vi "Requests.vi"(8 "error in (no error)":errorcluster, 9 "write enable":bool=TRUE, 11 "ICPCON ET7028 in":refnum<class "ICPCON ET-7028.lvclass">) -> (0 "error out":errorcluster, 3 "ICPCON ET7028 out":refnum<class "ICPCON ET-7028.lvclass">)   [LabVIEW 2021, in "ICPCON ET-7028.lvclass"]
uses:
  ICPCON ET-7028.lvclass
  D:/my_projects/projects/Algorithms/Labview/21/Modbus_v121c/Network Protocol/MB/Modbus Master CR.lvclass
  D:/my_projects/projects/Algorithms/Labview/21/Modbus_v121c/Network Protocol/Network Master/Network Master.lvclass
  MB/Modbus Master CR.lvclass/Modbus Master CR.ctl
  Modbus Data Unit/Modbus Data Unit.lvclass/Modbus Data Unit.ctl
  Network Protocol.lvclass/Network Protocol.ctl
  Network Master/Network Master.lvclass/Network Master.ctl
  Master Function Definition/Read Holding Registers Request.vi
  Master Function Definition/Read Holding Registers Response.vi
  Network Master/Read write Master.vi
  Master Function Definition/Write Multiple Registers Request.vi
  Master Function Definition/Function data mismatch error.vi
  Master Function Definition/Write Multiple Registers Response.vi
  Modbus Data Unit/Construct PDU.vi
  Utility/Bytes to U16s.vi
  Master Function Definition/Function code mismatch error.vi
  Data Model/Error Generator.vi
  Modbus Data Unit/Deconstruct PDU.vi
  Read Transmission Data Unit.vi
  Utility/U16s to Bytes.vi
  Network Master/Network Master.lvclass
  D:/my_projects/projects/Algorithms/Labview/21/Modbus_v121c/Network Protocol/Network Protocol.lvclass
  Modbus Data Unit/Modbus Data Unit.lvclass
  Data Model/Device Data Model.lvclass
  Transmission Data Unit/Transmission Data Unit.lvclass
  MB/Modbus Master CR.lvclass
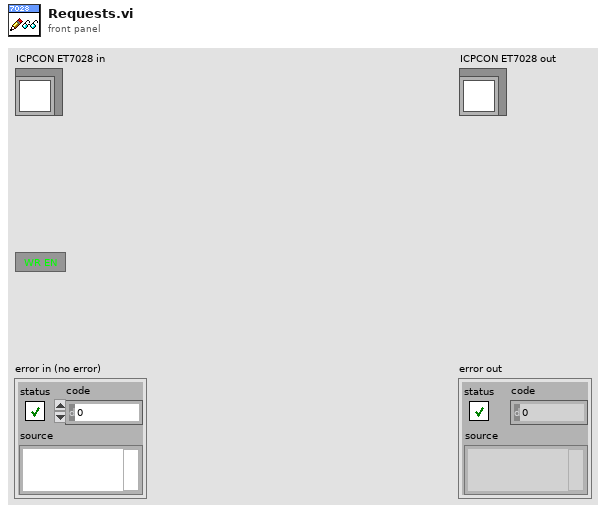
[diagram p1: front panel]
types:
  T1 = typedef "Modbus Master CR.lvclass/N channel.ctl" = cluster{"N DI channel":u16, "N DO channel":u16, "N AI channel":u16, "N AO channel":u16}
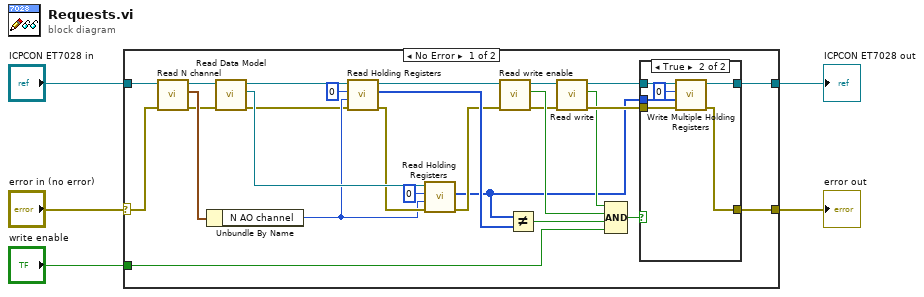
[diagram p0: block diagram]
diagram:
  n1 = case shown="No Error" "error in (no error)" {
    selector: "error in (no error)" -> [w27 w42]
    tunnel: [w31 w42] -> w3
    tunnel: [w7 w41] -> w4
    tunnel: "ICPCON ET7028 in" -> [w29 w41]
    tunnel: "write enable" -> [w23 _]
    frame No Error {
      n2 = call "Read N channel.vi"("error in (no error)"=w27, "MB_v2 in"=w29) -> ("error out"=w26:errorcluster, "N channel"=w30:T1, "MB_v2 out"=w28:refnum<class "ICPCON ET-7028.lvclass">)  [unwired: 7 in]
      n3 = Unbundle By Name(w30) -> ("N AO channel"=w12:u16)
      n4 = call "Read Data Model.vi"("error in (no error)"=w26, "MB_TCP in"=w28) -> ("error out"=w10:errorcluster, "Data Model"=w17:refnum<class "Device Data Model.lvclass">, "MB_TCP out"=w11:refnum<class "ICPCON ET-7028.lvclass">)  [unwired: 7 in]
      n5 = call "Read Holding Registers.vi"("error in (no error)"=w10, "number of holding registers"=w12, "starting address"=u16 0, "Modbus master in"=w11) -> ("error out"=w13:errorcluster, "register values"=w15:u16[], "Modbus master out"=w9:refnum<class "ICPCON ET-7028.lvclass">)  [unwired: 5 in]
      n6 = call-dynamic "Read Holding Registers.vi"("error in"=w13, "number of registers"=w12, "starting address"=u16 0, "device data model in"=w17) -> ("error out"=w14:errorcluster, "data"=w6:u16[])  [unwired: 5 in, 1 out]
      n7 = call "Read write enable.vi"("error in (no error)"=w14, "MB in"=w9) -> ("error out"=w21:errorcluster, "write enable"=w24:bool, "MB out"=w22:refnum<class "ICPCON ET-7028.lvclass">)  [unwired: 7 in]
      n8 = Not Equal?(x=w6, y=w15) -> (x != y?=w25:bool)
      n9 = call "Read write.vi"("error in (no error)"=w21, "MB in"=w22) -> ("error out"=w20:errorcluster, "Write"=w19:bool, "MB out"=w8:refnum<class "ICPCON ET-7028.lvclass">)  [unwired: 7 in]
      n10 = Compound Arithmetic op=AND(w19, w24, w25, w23) -> (w32:bool)
      n11 = case shown="True" w32 {
        tunnel: w20 -> [w34 w38]
        tunnel: [w34 w36] -> w31
        tunnel: w6 -> [_ w37]
        tunnel: w8 -> [w33 w39]
        tunnel: [w33 w35] -> w7
        frame False {
        }
        frame True {
          n12 = call "Write Multiple Holding Registers.vi"("error in (no error)"=w38, "holding register values"=w37, "starting address"=u16 0, "Modbus master in"=w39) -> ("error out"=w36:errorcluster, "Modbus master out"=w35:refnum<class "ICPCON ET-7028.lvclass">)  [unwired: 6 in]
        }
      }
    }
    frame Error {
    }
  }
  "error out" <- w3
  "ICPCON ET7028 out" <- w4
